vi "ReferencedVariables_ReadWriteReferencedVariable_4x4x4_Singleton.vi"(8 "error in (no error)":errorcluster, 10 "ReplaceWithtypeDef":dbl) -> (0 "error out":errorcluster)   [LabVIEW 2020]
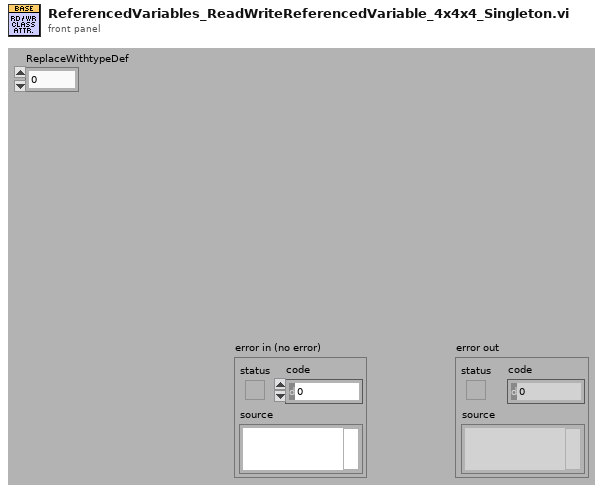
[diagram p1: front panel]
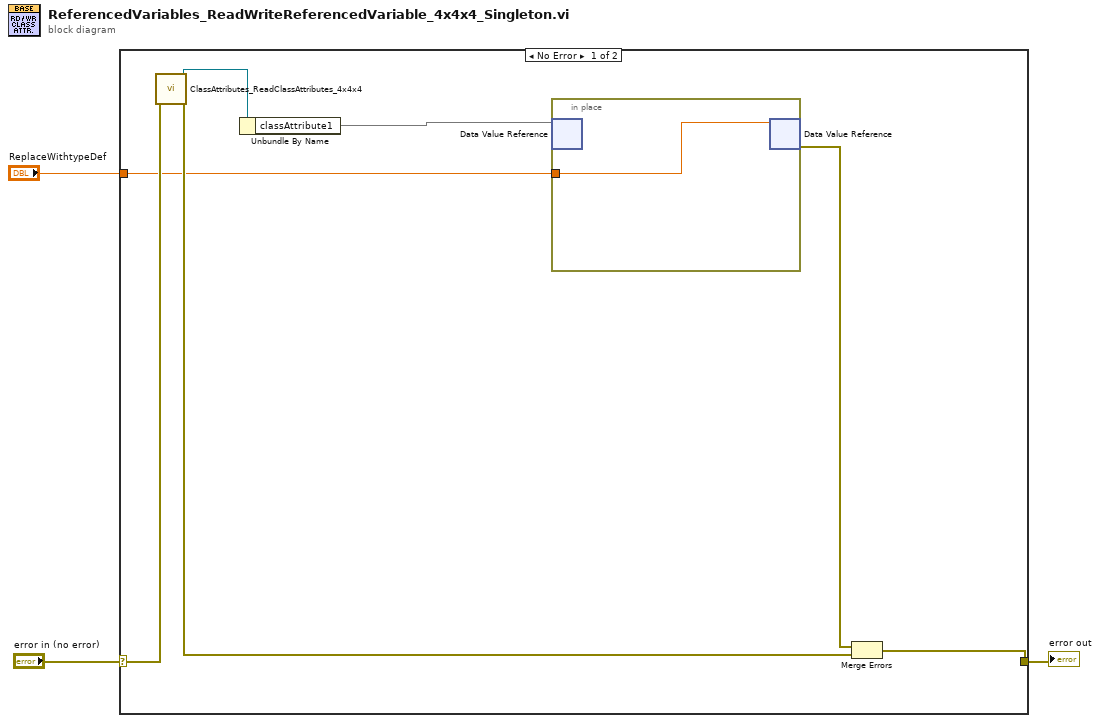
[diagram p0: block diagram]
diagram:
  n1 = case shown="No Error" "error in (no error)" {
    selector: "error in (no error)" -> [w8 w12]
    tunnel: [w9 w12] -> w2
    tunnel: "ReplaceWithtypeDef" -> [w4 _]
    frame No Error {
      n2 = call <resource>:"ClassAttributes_ReadClassAttributes_4x4x4.vi"("error in (no error)"=w8) -> ("error out"=w5:errorcluster, "reference out"=w7:refnum<class>)  [unwired: 9 in]
      n3 = Unbundle By Name(w7) -> ("classAttribute1"=w6)
      n4 = in-place {
        in-place-border: w4 -> [w11]
        n5 = in-place-dvr #1(w6) -> ()  [unwired: 2 out]
        n6 = in-place-dvr #1(w11) -> (w10:errorcluster)  [unwired: 1 out]
      }
      n7 = Merge Errors(w10, w5) -> (w9:errorcluster)
    }
    frame Error {
    }
  }
  "error out" <- w2
